vi "tmp_toml_example.vi"() -> ()   [LabVIEW 2017]
uses:
  b87011d9-6f61-4e8a-a239-e3f8ce84dcb3.vi
  f8c66d1a-572e-43cb-98dd-acf2abf72035.vi
  52bd2232-900c-45fb-b2bc-76806f9ad0f5.vi
  tmp_toml_lock_acquire.vi
  tmp_toml_lock_release.vi
  <vilib>/Utility/error.llb/Clear Errors.vi
  tmp_toml_fg.vi
  <vilib>/Utility/file.llb/Application Directory.vi
panel:
  out "exists_get":bool
  out "value_get":i32
  out "exists_set":bool
  out "exists_sections":bool
  out "sections":string[](array[string])
  out "text_file":string
  out "exists_file":bool
  out "files loaded":path[](array[path])
  out "exists_setdefault":bool
  out "value_setdefault":i32
  out "error out":errorcluster
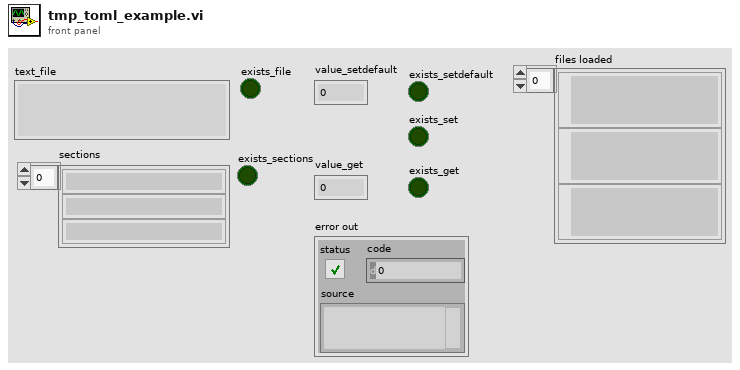
[diagram p1: front panel]
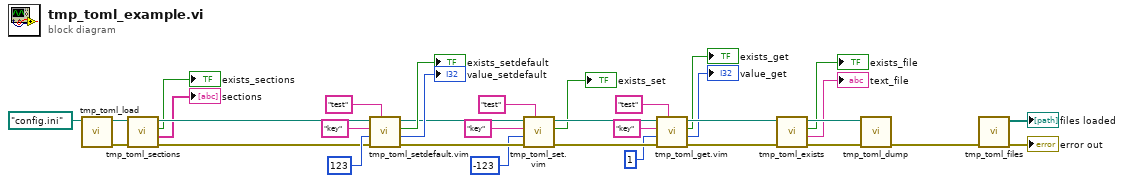
[diagram p0: block diagram]
diagram:
  n1 = call "tmp_toml_load.vi"("path in"=path "config.ini") -> ("error out"=w22:errorcluster, "path out"=w20:path)  [unwired: 8 in, 1 out]
  n2 = call "tmp_toml_sections.vi"("error in (no error)"=w22, "path in"=w20) -> ("error out"=w21:errorcluster, "sections"=→"sections":string[], "file exists"=→"exists_sections":bool, "path out"=w19:path)  [unwired: 6 in]
  n3 = call "tmp_toml_setdefault.vim"("section"="test", "error in (no error)"=w21, "default"=123, "key"="key", "path in"=w19) -> ("error out"=w15:errorcluster, "value"=→"value_setdefault":i32, "key exists"=→"exists_setdefault":bool, "path out"=w16:path)  [unwired: 3 in]
  n4 = call "tmp_toml_set.vim"("section"="test", "error in (no error)"=w15, "value"=-123, "key"="key", "path in"=w16) -> ("error out"=w10:errorcluster, "key exists"=→"exists_set":bool, "path out"=w14:path)  [unwired: 4 in]
  n5 = call "tmp_toml_get.vim"("section"="test", "error in (no error)"=w10, "default"=1, "key"="key", "path in"=w14) -> ("error out"=w6:errorcluster, "value"=→"value_get":i32, "key exists"=→"exists_get":bool, "path out"=w5:path)  [unwired: 3 in]
  n6 = call "tmp_toml_exists.vi"("error in (no error)"=w6, "path in"=w5) -> ("error out"=w26:errorcluster, "text"=→"text_file":string, "file exists"=→"exists_file":bool, "path out"=w27:path)  [unwired: 6 in]
  n7 = call "tmp_toml_dump.vi"("error in (no error)"=w26, "path in"=w27) -> ("error out"=w25:errorcluster)  [unwired: 7 in, 2 out]
  n8 = call "tmp_toml_files.vi"("error in (no error)"=w25) -> ("error out"=→"error out":errorcluster, "files loaded"=→"files loaded":path[])  [unwired: 9 in]
